vi "ui_DataLog Show Big String.vi"(0 "title":string, 7 "string to show":string) -> ()   [LabVIEW 2012]
doc: "This dialog shows a big string using a selectable display mode."
uses:
  typedefs/t_DataLog Show Big String States.ctl
panel:
  in  "display mode":u16(ring) items=["normal", "backslash codes", "hexadecimal"]
  out "string":string
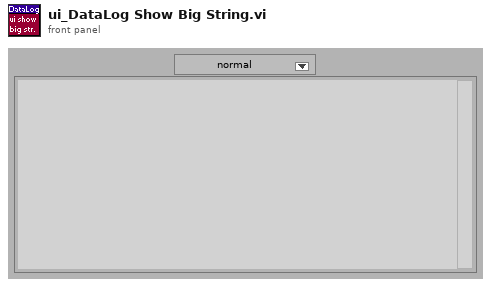
[diagram p1: front panel]
types:
  T1 = typedef "t_DataLog Show Big String States.ctl" = enum16{"empty queue", "set style", "initialize", "stop"}
  T2 = typedef "eventvkey.ctl" = enum16{"ASCII", "Enter", "Return", "Shift", "Ctrl", "Alt", "Cmd", "Opt", "Caps", "NumLock", "Clear", "Break", "Up", "Down", "Left", "Right", "Insert", "Delete", "Home", "End", "PageUp", "PageDown", "Escape", "Help", "Pause", "ScrollLock", "F1", "F2", "F3", "F4", "F5", "F6", "F7", "F8", "F9", "F10", "F11", "F12", "F13", "F14", "F15", "F16", "F17", "F18", "F19", "F20", "F21", "F22", "F23", "F24", "Play", "VolumeUp", "VolumeDown", "Mute", "Two Byte Char"}
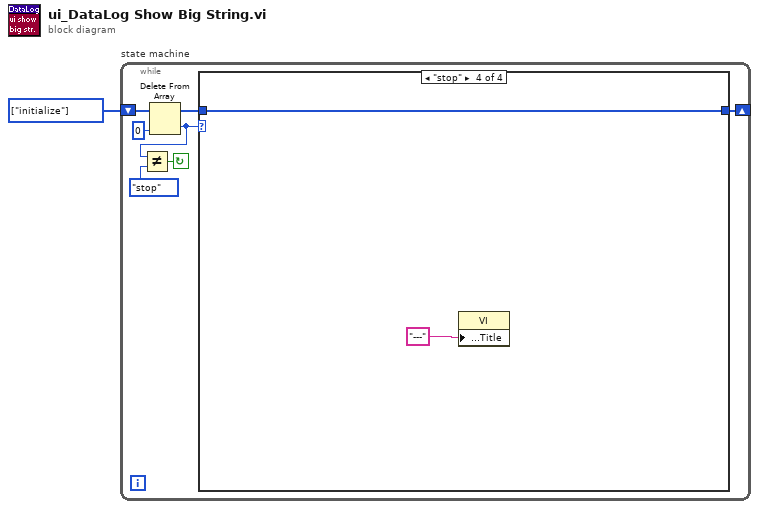
[diagram p0: block diagram]
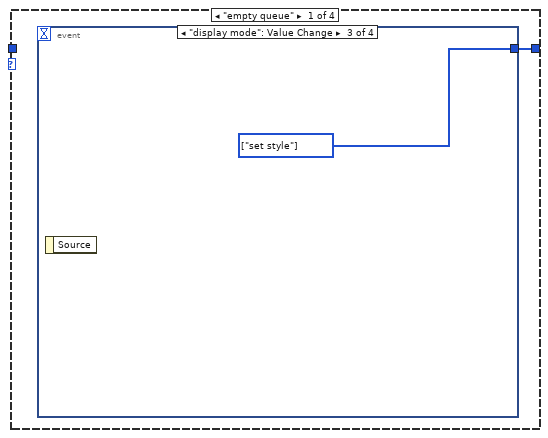
[diagram p2: hidden frame]
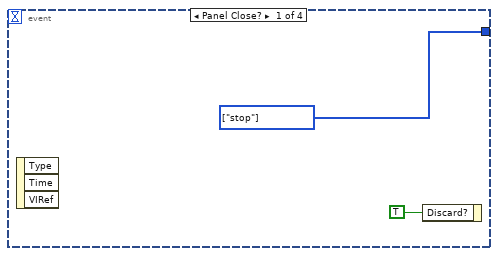
[diagram p3: hidden frame]
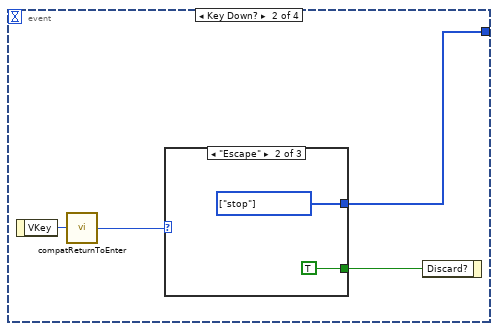
[diagram p4: hidden frame]
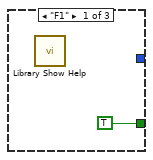
[diagram p5: hidden frame]
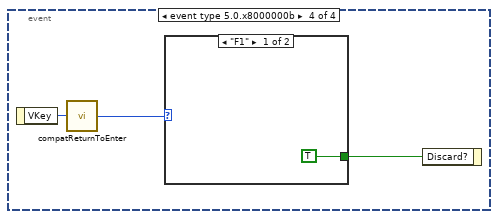
[diagram p7: hidden frame]
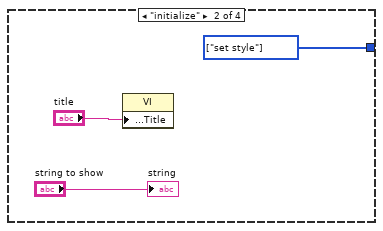
[diagram p9: hidden frame]
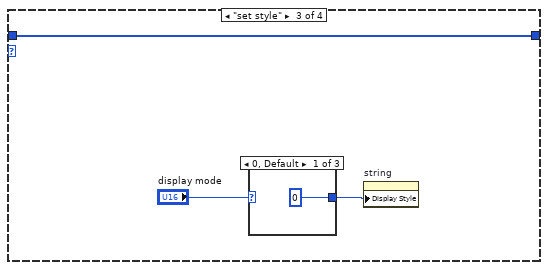
[diagram p10: hidden frame]
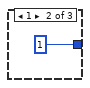
[diagram p11: hidden frame]
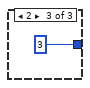
[diagram p12: hidden frame]
diagram:
  w1 = T1[] [enum."initialize"] items=["empty queue", "set style", "initialize", "stop"] ("Array Constant")
  n1 = while "state machine" {
    shift-left: w1 -> [w5]
    shift-right: [w8] -> _
    stop <- w7 continue-if-true
    n2 = Delete From Array(array=w5, index=0) -> (deleted portion=w3:T1, array with subset deleted=w4:T1[])  [unwired: 1 in]
    n3 = Not Equal?(x=w3, y=t_DataLog_Show_Big_String_States."stop" ("states")) -> (x != y?=w7:bool)
    n4 = case "Case" shown="\"stop\"" w3 {
      tunnel: [w9 w24 w29 w34] -> w8
      tunnel: w4 -> [_ _ w29 w34]
      frame "empty queue" {
        n5 = event shown="[2] \"display mode\": Value Change" {
          selector: _ -> [_ _ _ _]
          dyn-events: _ -> [_ _ _ _]
          timeout: _ -> [_ _ _ _]
          tunnel: [w11 w13 w19 _] -> w9
          event Panel Close? {
            w11 = T1[] [enum."stop"] items=["empty queue", "set style", "initialize", "stop"] ("Array Constant")
            n6 = event-data() -> ()  [unwired: 1 in, 3 out]
            n7 = event-data("Discard?"=TRUE) -> ()  [unwired: 1 in, 1 out]
          }
          event Key Down? {
            n8 = event-data() -> ("VKey"=w12:T2)  [unwired: 1 in]
            n9 = call <vilib>:"compatReturnToEnter.vi"("VKey"=w12) -> ("VKey"=w15:T2)
            n10 = case shown="\"Escape\"" w15 {
              tunnel: [TRUE ("Discard?") TRUE ("Discard?") _] -> w14
              tunnel: [_ w17 _] -> w13
              frame "F1" {
                n11 = call "Library Show Help.vi"() -> ()  [unwired: 1 in]
              }
              frame "Escape" {
                w17 = T1[] [enum."stop"] items=["empty queue", "set style", "initialize", "stop"] ("Array Constant")
              }
              frame Default {
              }
            }
            n12 = event-data("Discard?"=w14) -> ()  [unwired: 1 in, 1 out]
          }
          event "display mode": Value Change {
            w19 = T1[] [enum."set style"] items=["empty queue", "set style", "initialize", "stop"] ("Array Constant")
            n13 = event-data() -> ()  [unwired: 1 in, 1 out]
          }
          event event type 5.0.x8000000b {
            n14 = event-data() -> ("VKey"=w20:T2)  [unwired: 1 in]
            n15 = call <vilib>:"compatReturnToEnter.vi"("VKey"=w20) -> ("VKey"=w22:T2)
            n16 = case shown="\"F1\"" w22 {
              tunnel: [TRUE ("Discard?") _] -> w21
              frame "F1" {
              }
              frame Default {
              }
            }
            n17 = event-data("Discard?"=w21) -> ()  [unwired: 1 in, 1 out]
          }
        }
      }
      frame "initialize" {
        w24 = T1[] [enum."set style"] items=["empty queue", "set style", "initialize", "stop"] ("Array Constant")
        n18 = property class="VI"("Front Panel Window:Title"="title") -> ()  [unwired: 2 in, 2 out]
        "string" <- "string to show"
      }
      frame "set style" {
        n19 = case shown="0, Default" "display mode" {
          tunnel: [u32 0 ("Display Style") u32 1 ("Display Style") u32 3 ("Display Style")] -> w27
          frame 0, Default {
          }
          frame 1 {
          }
          frame 2 {
          }
        }
        n20 = property on="string" class="Str"("Display Style"=w27) -> ()  [unwired: 2 in, 2 out]
      }
      frame "stop" {
        n21 = property class="VI"("Front Panel Window:Title"="---") -> ()  [unwired: 2 in, 2 out]
      }
    }
  }
